vi "_Get SheetData.vi"(8 "error in":errorcluster, 11 "Worksheet in":refnum<k24>) -> (0 "error out":errorcluster, 2 "SheetData":refnum<k24>, 3 "Worksheet out":refnum<k24>)   [LabVIEW 2021, in "Open Xml.lvlib"]
uses:
  Open Xml.lvlib
  D:/git/Open-Xml-LabVIEW/dll/DocumentFormat.OpenXml.dll
  dll/DocumentFormat.OpenXml.dll
  D:/git/Open-Xml-LabVIEW/dll/DocumentFormat.OpenXml.Framework.dll
  dll/DocumentFormat.OpenXml.Framework.dll
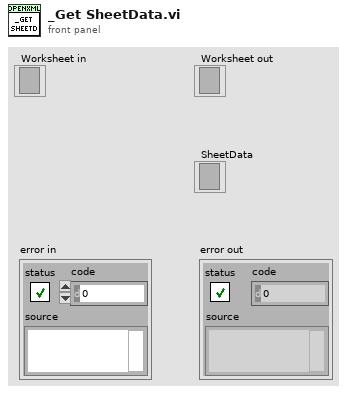
[diagram p1: front panel]
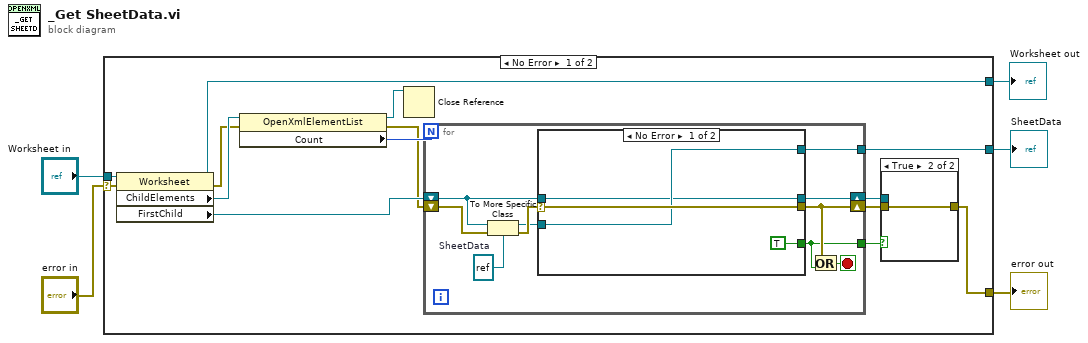
[diagram p0: block diagram]
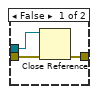
[diagram p2: hidden frame]
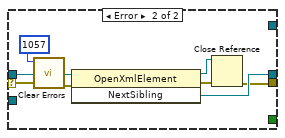
[diagram p3: hidden frame]
diagram:
  n1 = case shown="No Error" "error in" {
    selector: "error in" -> [w18 w47]
    tunnel: "Worksheet in" -> [w19 w46]
    tunnel: [w17 _] -> w3
    tunnel: [w8 w47] -> w2
    tunnel: [w11 w46] -> w1
    frame No Error {
      n2 = property class="Worksheet"(reference=w19, error in=w18) -> (reference out=w11:refnum<k24>, error out=w12:errorcluster, "ChildElements"=w14:refnum<k24>, "FirstChild"=w15:refnum<k24>)
      n3 = property class="OpenXmlElementList"(reference=w14, error in=w12) -> (reference out=w9:refnum<k24>, error out=w10:errorcluster, "Count"=w13:i32)
      n4 = Close Reference(reference=w9) -> ()  [unwired: 1 in, 1 out]
      n5 = for "Find SheetData" {
        N: w13 -> [_]
        shift-right: [w28] -> w7
        shift-left: w15 -> [w31]
        tunnel: [w29] -> w17
        shift-right: [w25] -> w16
        shift-left: w10 -> [w27]
        tunnel: [w24] -> w6
        stop <- w26 stop-if-true
        w32 = refnum<k24> refnum  # SheetData
        n6 = To More Specific Class(target class=w32, reference=w31, error in=w27) -> (specific class reference=w30:refnum<k24>, error out=w33:errorcluster)
        n7 = case shown="No Error" w33 {
          selector: w33 -> [w37 w42]
          tunnel: [w37 w38] -> w25
          tunnel: [w34 w45] -> w28
          tunnel: [TRUE _] -> w24
          tunnel: w31 -> [w34 w44]
          tunnel: w30 -> [w35 _]
          tunnel: [w35 _] -> w29
          frame No Error {
          }
          frame Error {
            n8 = call <vilib>:"Clear Errors.vi"("error in (no error)"=w42, "specific error code to clear (0: all)"=1057) -> ("error out"=w41:errorcluster)  [unwired: 4 in, 1 out]
            n9 = invoke class="OpenXmlElement" method="NextSibling"(reference=w44, error in=w41) -> (reference out=w43:refnum<k24>, error out=w39:errorcluster, "NextSibling"=w45:refnum<k24>)  [unwired: 1 in]
            n10 = Close Reference(reference=w43, error in (no error)=w39) -> (error out=w38:errorcluster)
          }
        }
        n11 = Or(x=w25, y=w24) -> (x .or. y?=w26:bool)
      }
      n12 = case shown="True" w6 {
        tunnel: w16 -> [w22 w23]
        tunnel: [w21 w23] -> w8
        tunnel: w7 -> [w20 _]
        frame False {
          n13 = Close Reference(reference=w20, error in (no error)=w22) -> (error out=w21:errorcluster)
        }
        frame True {
        }
      }
    }
    frame Error {
    }
  }
  "error out" <- w2
  "SheetData" <- w3
  "Worksheet out" <- w1
